vi "获取合法节点列表.vi"(11 "节点引用数组":refnum<vi>[](array[refnum])) -> (3 "节点列表":T1(array[cluster]))   [LabVIEW 2019]
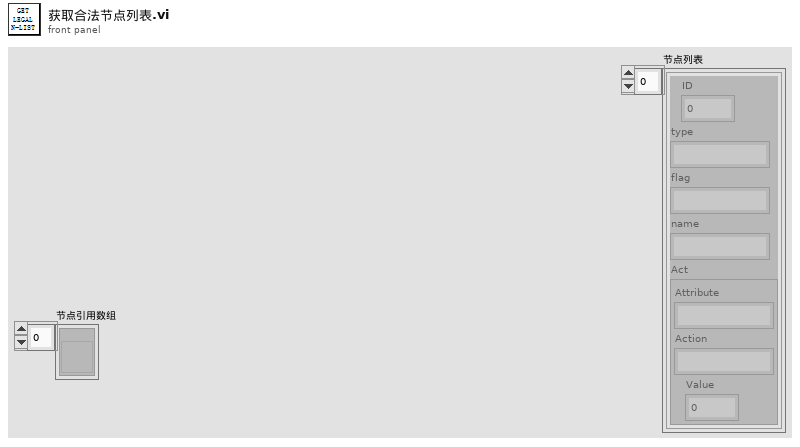
[diagram p1: front panel]
types:
  T1 = cluster{"ID":u8, "type":string, "flag":string, "name":string, "Act":cluster{"Attribute":string, "Action":string, "Value":dbl}}[]
  T2 = cluster{"ID":u8, "type":string, "flag":string, "name":string, "Act":cluster{"Attribute":string, "Action":string, "Value":dbl}}
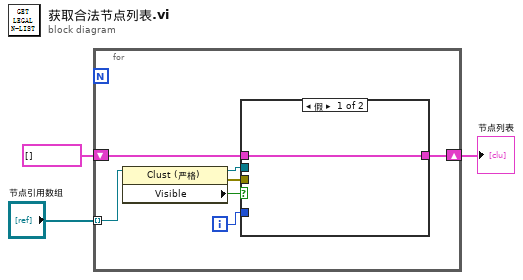
[diagram p0: block diagram]
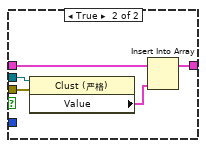
[diagram p2: hidden frame]
diagram:
  n1 = for {
    tunnel: "节点引用数组" -> [w10] mode=indexing
    shift-right: [w8] -> w1
    shift-left: T1 [] -> [w7]
    i -> [w9]
    n2 = property class="Clust (严格)"(reference=w10) -> (reference out=w5:refnum<vi>, error out=w4:errorcluster, "Visible"=w6:bool)  [unwired: 1 in]
    n3 = case shown="假" w6 {
      tunnel: w9 -> [_ _]
      tunnel: [w11 w15] -> w8
      tunnel: w7 -> [w11 w14]
      tunnel: w5 -> [_ w13]
      tunnel: w4 -> [_ w12]
      frame False {
      }
      frame True {
        n4 = property class="Clust (严格)"(reference=w13, error in=w12) -> ("Value"=w16:T2)  [unwired: 2 out]
        n5 = Insert Into Array(array=w14, new element=w16) -> (w15:T1)  [unwired: 1 in]
      }
    }
  }
  "节点列表" <- w1
